vi "create subscription cancel message.vi"(11 "pattern":string) -> (3 "message":refnum<class "communicator message.lvclass">)   [LabVIEW 2015, in "publisher.lvclass"]
uses:
  publisher.lvclass
  message/communicator message.lvclass
  message/communicator message.lvclass/communicator message.ctl
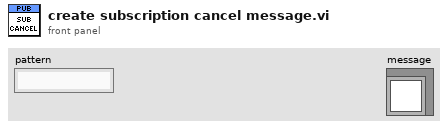
[diagram p1: front panel]
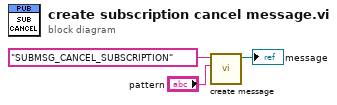
[diagram p0: block diagram]
diagram:
  n1 = call "create message.vi"("data"="pattern", "ID"="SUBMSG_CANCEL_SUBSCRIPTION") -> ("message"=→"message":refnum<class "communicator message.lvclass">)  [unwired: 9 in]
